vi "checkFinishNormalGamePlay.vi"(7 "OffensiveTeam":refnum<class "Ally.lvclass">, 8 "error in (no error)":errorcluster, 9 "last command_interpreted":T1, 10 "Game":refnum<class "Game.lvclass">, 11 "NormalGamePlay in":refnum<class "NormalGamePlay.lvclass">) -> (0 "error out":errorcluster, 1 "OffensiveTeam out":refnum<class "Ally.lvclass">, 2 "finish?":bool, 3 "NormalGamePlay out":refnum<class "NormalGamePlay.lvclass">)   [LabVIEW 2021, in "NormalGamePlay.lvclass"]
uses:
  NormalGamePlay.lvclass
  Game_class/Game.lvclass
  Referee_class/command_interpreted.ctl
  Ally_class/Ally.lvclass
  Utilities_class/Utilities.lvclass
  Game_class/Game.lvclass/Game.ctl
  Referee_class/Referee.lvclass/Referee.ctl
  Events_class/Events.lvclass/Events.ctl
  Object_class/Object.lvclass/Object.ctl
  Game_class/Read Referee.vi
  Game_class/Read EventsRef.vi
  Game_class/Read BallRef.vi
  Object_class/Read x.vi
  Object_class/Read y.vi
  Events_class/Read enemy_ball_possesion.vi
  Events_class/Read ball_out.vi
  Referee_class/Read command_interpreted.vi
  Ball_class/Ball.lvclass
  D:/RoboIme/horie/SSL_AI/Object_class/Object.lvclass
  Referee_class/Referee.lvclass
  Events_class/Events.lvclass
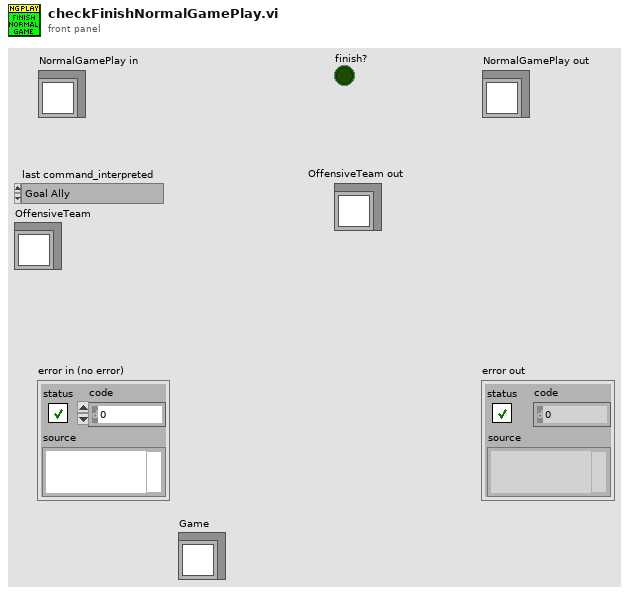
[diagram p1: front panel]
types:
  T1 = typedef "command_interpreted.ctl" = enum16{"Goal Ally", "Goal Enemy", "Ball Placement Enemy", "Ball Placement Ally", "Normal Half Time", "Extra Time  Break", "Extra Half Time", "None", "Post Game", "PKA Normal Start", "Prepare Kickoff Ally", "PKE Normal Start", "Prepare Kickoff Enemy", "Force Start", "Halt", "Timeout", "Prepare Penalty Ally", "Prepare Penalty Enemy", "PPA NormalStart", "PPE Normal Start", "Indirect Free Ally", "Direct Free Enemy", "Direct Free Ally", "Indirect Free Enemy", "Stop"}
  T2 = typedef "OffensivePlay.ctl" = enum16{"5RobotsPassGamePlay", "5PreparePassGame", "5RobotsKeeperGame", "KeeperPassToStriker", "5RobotsNormalGamePlay", "PrepareKeeperPass", "ACBPass", "ABCPass", "PrepareTriplePass", "TableWithStriker", "TableWith2ndStrikerPlay", "PrepareDoublePass", "PrepareRollToPass", "SimplePass", "PreparePass", "PassToStriker", "BallOutOfField", "PassTo2ndStriker", "StopOffensive", "Prepare Penalty Enemy", "EnemyPossessionAtEnemyField", "EnemyPossesionAtOurField", "TestPlay", "PreparePenaltyAlly", "KickPenaltyAlly", "PrepareKickoffAlly", "PrepareKickoffEnemy", "IndirectEnemy", "DirectEnemy", "PreparePassInGame1", "NormalGame", "DirectKick", "Pass", "Halt", "Timeout", "PassPlay", "PenaltyEnemy"}
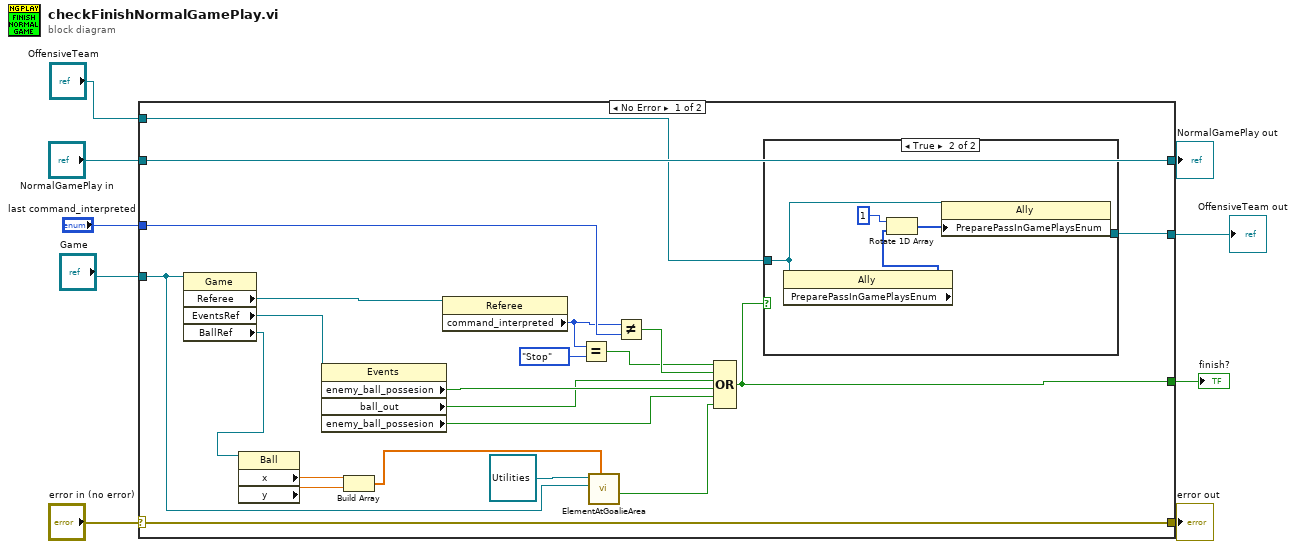
[diagram p0: block diagram]
diagram:
  n1 = case shown="No Error" "error in (no error)" {
    selector: "error in (no error)" -> [w30 w39]
    tunnel: [w30 w39] -> w8
    tunnel: [w31 w38] -> w6
    tunnel: "NormalGamePlay in" -> [w31 w38]
    tunnel: "Game" -> [w11 _]
    tunnel: [w19 _] -> w4
    tunnel: "last command_interpreted" -> [w23 _]
    tunnel: "OffensiveTeam" -> [w18 _]
    tunnel: [w17 _] -> w1
    frame No Error {
      n2 = property class="Game"(reference=w11) -> ("Referee"=w29:refnum<class "Referee.lvclass">, "EventsRef"=w28:refnum<class "Events.lvclass">, "BallRef"=w15:refnum<class "Ball.lvclass">)  [unwired: 1 in, 2 out]
      n3 = property class="Ball"(reference=w15) -> ("x"=w14:dbl, "y"=w13:dbl)  [unwired: 1 in, 2 out]
      n4 = property class="Events"(reference=w28) -> ("enemy_ball_possesion"=w26:bool, "ball_out"=w25:bool, "enemy_ball_possesion"=w24:bool)  [unwired: 1 in, 2 out]
      n5 = Build Array(w14, w13) -> (w12:dbl[])
      n6 = property class="Referee"(reference=w29) -> ("command_interpreted"=w22:T1)  [unwired: 1 in, 2 out]
      n7 = Equal?(x=w22, y=command_interpreted."Stop") -> (x = y?=w20:bool)
      n8 = call "ElementAtGoalieArea.vi"("Elemento pos."=w12, "Game"=w11, "Utilities in"=refnum<class "Utilities.lvclass"> refnum) -> ("Element at our goalkeeper area ?"=w10:bool)  [unwired: 4 in, 4 out]
      n9 = Not Equal?(x=w22, y=w23) -> (x != y?=w27:bool)
      n10 = Compound Arithmetic op=OR(w20, w27, w25, w26, w24, w10) -> (w19:bool)
      n11 = case shown="True" w19 {
        tunnel: [w32 w35] -> w17
        tunnel: w18 -> [w32 w34]
        frame False {
        }
        frame True {
          n12 = property class="Ally"(reference=w34) -> ("PreparePassInGamePlaysEnum"=w33:T2[])  [unwired: 1 in, 2 out]
          n13 = Rotate 1D Array(1:w33, 2:1 ("n")) -> (0:w36:T2[])
          n14 = property class="Ally"(reference=w34, "PreparePassInGamePlaysEnum"=w36) -> (reference out=w35:refnum<class "Ally.lvclass">)  [unwired: 1 in, 1 out]
        }
      }
    }
    frame Error {
    }
  }
  "error out" <- w8
  "NormalGamePlay out" <- w6
  "finish?" <- w4
  "OffensiveTeam out" <- w1
